vi "GetDisplayName.vi"(8 "No Error":errorcluster, 11 "Display ID":T1) -> (0 "Error Out":errorcluster, 3 "Displa Name":string)   [LabVIEW 2024, in "SDL3.lvlib" / "Video.lvlib"]
doc: "<B>Summary</B>\nGet the name of a display in UTF-8 encoding."
uses:
  Video.lvlib
  DisplayID--integer.ctl
  Lib/SDL3-32.dll
  Error/Error.lvlib
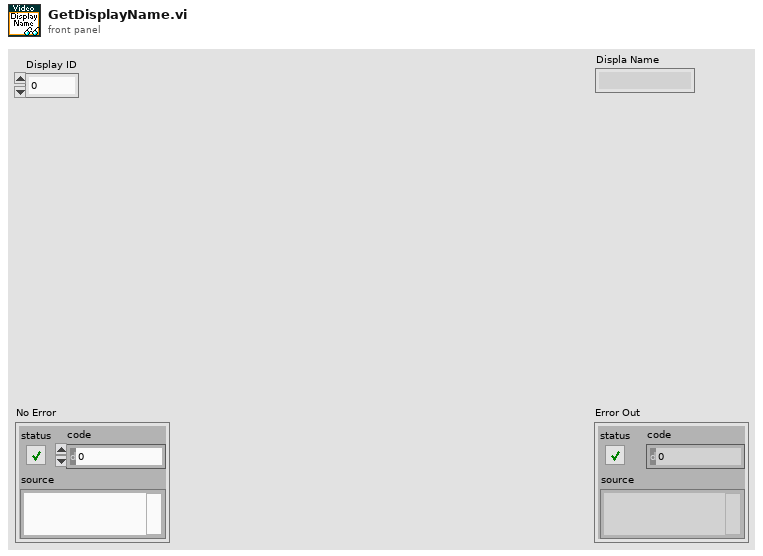
[diagram p1: front panel]
types:
  T1 = typedef "SDL3.lvlib/Video.lvlib/DisplayID--integer.ctl" = u32
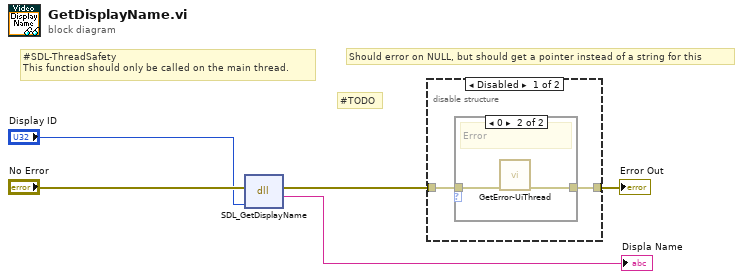
[diagram p0: block diagram]
diagram:
  # "#SDL-ThreadSafety\nThis function should only be called on the main thread."
  # "#TODO"
  # "Should error on NULL, but should get a pointer instead of a string for this"
  n1 = dll-call lib="C:/Users/Thomas/Documents/Projects/LV-SDL3/Lib/SDL3-*.*" fn="SDL_GetDisplayName"(error in="No Error", "displayID"="Display ID") -> (error out=w3:errorcluster, "return type"=→"Displa Name":string)  [unwired: 3 in, 1 out]
  n2 = disable-structure shown="Disabled" {
    disable-tunnel: [w7 w11] -> w4
    disable-tunnel: w3 -> [w6 w11]
    frame Disabled {
      n3 = case shown="0" {
        selector: _ -> [_ _]
        tunnel: w6 -> [w8 w10]
        tunnel: [w8 w9] -> w7
        frame Default {
          # "Ok"
        }
        frame 0 {
          # "Error"
          n4 = call "GetError-UiThread.vi"("No Error"=w10) -> ("error out"=w9:errorcluster)  [unwired: 10 in]
        }
      }
    }
    frame Enabled {
    }
  }
  "Error Out" <- w4
